vi "Post-Uninstall Custom Action.vi"(10 "Variant":variant) -> (0 "error out":errorcluster)   [LabVIEW 2014]
panel:
  out "dup file":path
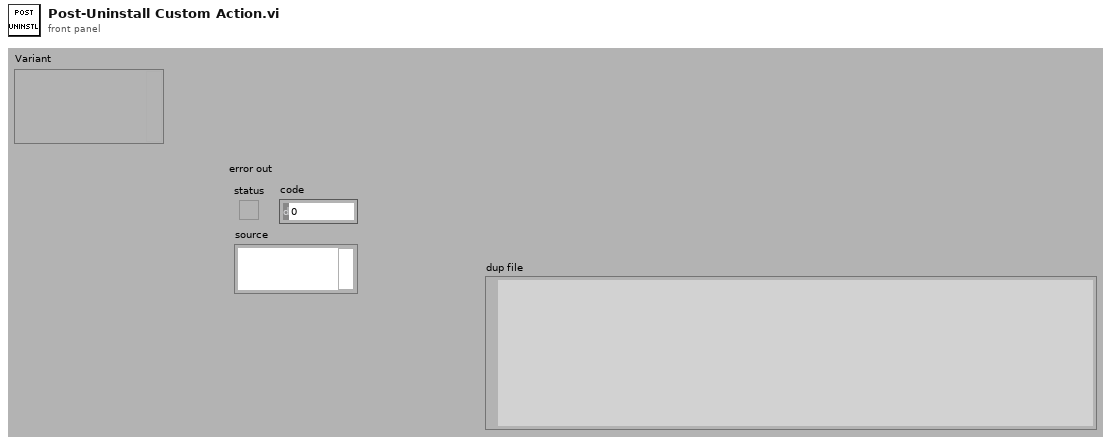
[diagram p1: front panel]
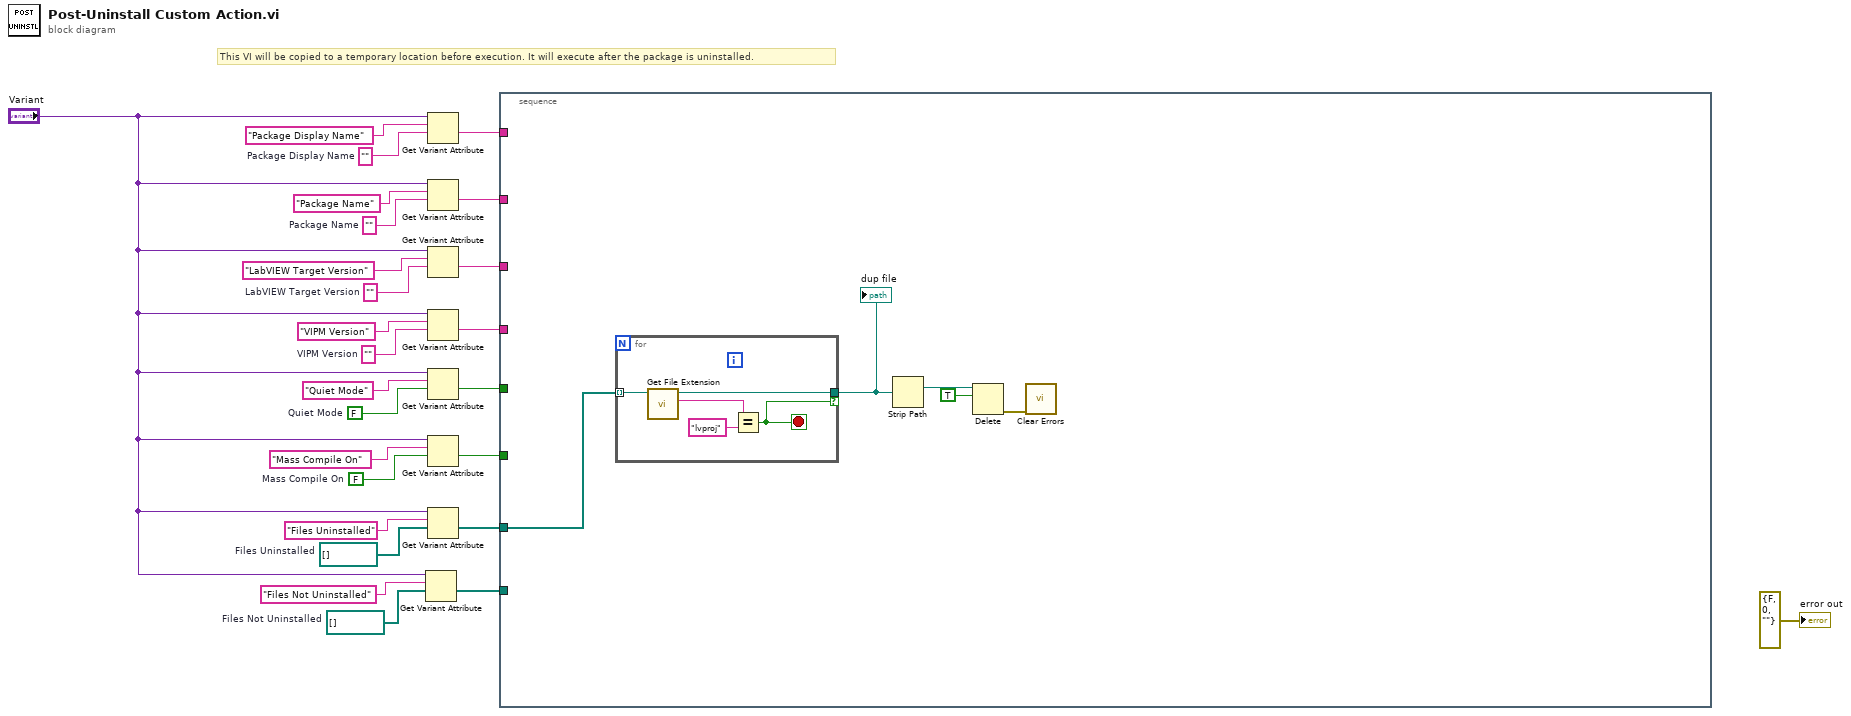
[diagram p0: block diagram]
diagram:
  w1 = path[] []  # Files Not Uninstalled
  w2 = path[] []  # Files Uninstalled
  w8 = FALSE  # Mass Compile On
  w9 = ""  # Package Display Name
  w16 = FALSE  # Quiet Mode
  w19 = ""  # VIPM Version
  w21 = ""  # LabVIEW Target Version
  w23 = ""  # Package Name
  # "This VI will be copied to a temporary location before execution. It will execute after the package is uninstalled."
  n1 = Get Variant Attribute(Variant="Variant", name="Files Not Uninstalled", default value (empty Variant)=w1) -> (value=w6:path[])  [unwired: 1 in, 3 out]
  n2 = Get Variant Attribute(Variant="Variant", name="Package Display Name", default value (empty Variant)=w9) -> (value=w15:string)  [unwired: 1 in, 3 out]
  n3 = Get Variant Attribute(Variant="Variant", name="Package Name", default value (empty Variant)=w23) -> (value=w14:string)  [unwired: 1 in, 3 out]
  n4 = Get Variant Attribute(Variant="Variant", name="LabVIEW Target Version", default value (empty Variant)=w21) -> (value=w13:string)  [unwired: 1 in, 3 out]
  n5 = Get Variant Attribute(Variant="Variant", name="VIPM Version", default value (empty Variant)=w19) -> (value=w12:string)  [unwired: 1 in, 3 out]
  n6 = Get Variant Attribute(Variant="Variant", name="Quiet Mode", default value (empty Variant)=w16) -> (value=w11:bool)  [unwired: 1 in, 3 out]
  n7 = Get Variant Attribute(Variant="Variant", name="Mass Compile On", default value (empty Variant)=w8) -> (value=w10:bool)  [unwired: 1 in, 3 out]
  n8 = Get Variant Attribute(Variant="Variant", name="Files Uninstalled", default value (empty Variant)=w2) -> (value=w5:path[])  [unwired: 1 in, 3 out]
  n9 = stacked-sequence {
    tunnel: w15 -> [_]
    tunnel: w14 -> [_]
    tunnel: w13 -> [_]
    tunnel: w12 -> [_]
    tunnel: w11 -> [_]
    tunnel: w10 -> [_]
    tunnel: w5 -> [w31]
    tunnel: w6 -> [_]
    frame #0 {
      n10 = for {
        tunnel: w31 -> [w36] mode=indexing
        tunnel: [w35] -> w30 if=w33
        stop <- w33 stop-if-true
        n11 = call <vilib>:"Get File Extension.vi"("file"=w36) -> ("lowercase file extension"=w32:string, "dup file"=w35:path)  [unwired: 7 in, 2 out]
        n12 = Equal?(x=w32, y="lvproj") -> (x = y?=w33:bool)
      }
      "dup file" <- w30
      n13 = Strip Path(path=w30) -> (stripped path=w29:path)  [unwired: 1 out]
      n14 = Delete(path (use dialog)=w29, entire hierarchy (F)=TRUE) -> (error out=w27:errorcluster)  [unwired: 3 in, 2 out]
      n15 = call <vilib>:"Clear Errors.vi"("error in (no error)"=w27) -> ()  [unwired: 6 in, 1 out]
    }
  }
  "error out" <- errorcluster {"status"=FALSE, "code"=0, "source"=""} ("error out")
